vi "TeleOP Reset Angle.vi"   [LabVIEW 2016]
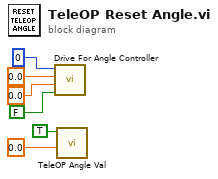
[diagram p0: block diagram]
diagram:
  n1 = call "Drive For Angle Controller.vi"("Vision"=FALSE, "Speed"=0.0, "Yaw"=0.0, "Iterations"=0) -> ()  [unwired: 5 in, 3 out]
  n2 = call "TeleOP Angle Val.vi"("TeleOP Angle (in)"=0.0 ("TeleOP Angle"), "Write"=TRUE) -> ()  [unwired: 9 in, 1 out]
